vi "PID.vi"(7 "PID Gains":cluster{"Kp":dbl, "Kd":dbl, "Ki":dbl}, 8 "Saturation":dbl, 9 "y(output)":i32, 10 "Reference":dbl) -> (3 "Control Input":dbl)   [LabVIEW 2018]
uses:
  Library/kevLib2011/Utilities/kCoerceFloat.vi
  Library/kevLib2011.lvlib
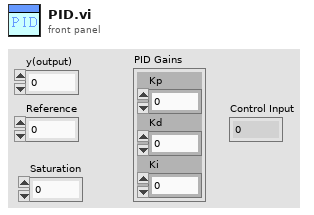
[diagram p1: front panel]
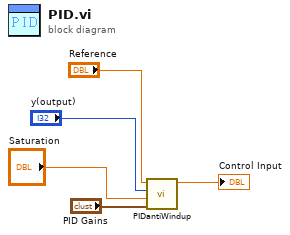
[diagram p0: block diagram]
diagram:
  n1 = call "PIDantiWindup.vi"("PID Gains"="PID Gains", "Saturation"="Saturation", "Position"="y(output)", "Reference"="Reference") -> ("control"=→"Control Input":dbl)  [unwired: 7 in]
